vi "Definition_3Wheel.vi"(8 "error in (no error)":errorcluster, 11 "KNR in":T1) -> (0 "error out":errorcluster, 3 "KNR out":T1)   [LabVIEW 2013]
uses:
  <userlib>/KNR OS 3.0 LabVIEW Toolkit/Type Definition/KNR3 Reference.ctl
  <userlib>/_FPGA Interface Advanced Tools/FPGA Interface Base/FPGA Interface Base.lvclass
  <userlib>/KNR OS 3.0 LabVIEW Toolkit/Type Definition/Resource.ctl
  <userlib>/KNR OS 3.0 LabVIEW Toolkit/Type Definition/DC Motor Port.ctl
  Global.vi
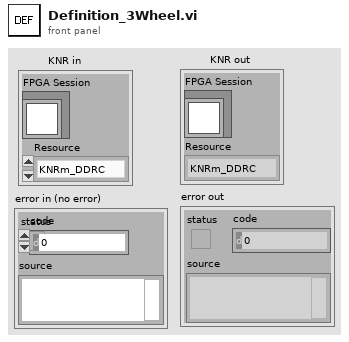
[diagram p1: front panel]
types:
  T1 = typedef "KNR3 Reference.ctl" = cluster{"FPGA Session":refnum<class "FPGA Interface Base.lvclass">, "Resource":T2}
  T2 = typedef "Resource.ctl" = enum16{"KNRm_DDRC", "KNRm_DDDD", "KNRm_DDDR", "KNRm_DDDC", "KNR"}
  T3 = typedef "DC Motor Port.ctl" = u16
  T4 = cluster{"Kvff":dbl, "Kpp":dbl, "Kvp":dbl, "Kvi":dbl, "Friction":dbl}
  T5 = cluster{"MM2DEG":dbl, "PLS2DEG":dbl, "Ts":dbl, "Tcnt":i32, "fs":i32, "Vmax":dbl, "Jmax":dbl, "N_Delay":i32, "C_port":T3, "KNRPLS":dbl}
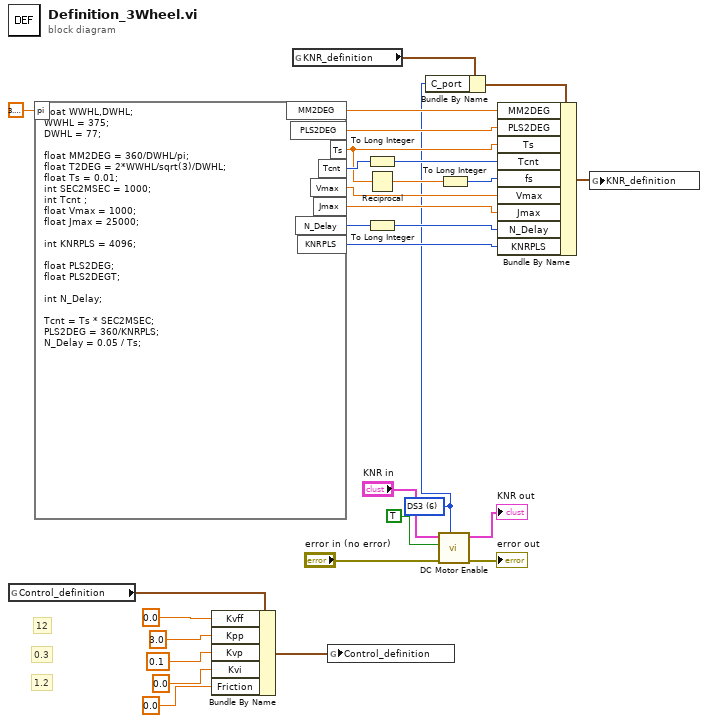
[diagram p0: block diagram]
diagram:
  w1 = T3 6 items=["DS1"=4, "DS2"=5, "DS3"=6, "DS4"=7] ("Port (DS1)")
  # "1.2"
  # "12"
  # "0.3"
  n1 = global read "Global.vi" "Control_definition"() -> (w29:T4)
  n2 = formula code="float WWHL,DWHL;\nWWHL = 375;\nDWHL = 77;\n\nfloat MM2DEG = 360/DWHL/pi;\nfloat T2DEG = 2*WWHL/sqrt(3)/DWHL;\nfloat Ts = 0.01;\nint SEC2MSEC = 1000;\nint Tcnt ;\nfloat Vmax = 1000;\nfloat Jmax = 25000;\n\nint KNRPLS = 4096;\n\nfloat PLS2DEG;\nfloat PLS2DEGT;\n\nint N_Delay;\n\nTcnt = Ts * SEC2MSEC;\nPLS2DEG = 360/KNRPLS;\nN_Delay = 0.05 / Ts;"("pi"=3.141592653589793) -> ("MM2DEG"=w10:dbl, "Tcnt"=w24:i32, "Ts"=w8:dbl, "Vmax"=w5:dbl, "Jmax"=w4:dbl, "N_Delay"=w23:i32, "PLS2DEG"=w9:dbl, "KNRPLS"=w2:i32)
  n3 = Bundle By Name(cluster=w29, "Kvff"=0.0 ("B_wheel.frict"), "Kpp"=3.0 ("input variable"), "Kvp"=0.1 ("input variable"), "Kvi"=0.0 ("input variable"), "Friction"=0.0 ("B_wheel.frict")) -> (w28:T4)
  n4 = global read "Global.vi" "KNR_definition"() -> (w27:T5)
  n5 = global write "Global.vi" "Control_definition"(w28) -> ()
  n6 = To Long Integer(number=w24) -> (32bit integer=w7:i32)
  n7 = Reciprocal(x=w8) -> (1/x=w26:dbl)
  n8 = To Long Integer(number=w23) -> (32bit integer=w3:i32)
  n9 = Bundle By Name(cluster=w27, "C_port"=w1) -> (w12:T5)
  n10 = call <userlib>:"DC Motor Enable.vi"("Port (DS1)"=w1, "error in (no error)"="error in (no error)", "Enable Motor(F)"=TRUE, "KNR in"="KNR in") -> ("error out"=→"error out":errorcluster, "KNR out"=→"KNR out":T1)  [unwired: 6 in]
  n11 = To Long Integer(number=w26) -> (32bit integer=w6:i32)
  n12 = Bundle By Name(cluster=w12, "MM2DEG"=w10, "PLS2DEG"=w9, "Ts"=w8, "Tcnt"=w7, "fs"=w6, "Vmax"=w5, "Jmax"=w4, "N_Delay"=w3, "KNRPLS"=w2) -> (w11:T5)
  n13 = global write "Global.vi" "KNR_definition"(w11) -> ()
